vi "HowdyArcade.vi"(7 "Negate Right input (true)":bool=TRUE, 9 "forward":dbl format="%#_13g", 10 "right":dbl format="%#_13g") -> (1 "right_wheel":dbl format="%#_13g", 2 "left_wheel":dbl format="%#_13g")   [LabVIEW 2019, in "DriveOld.lvlib" / "Drive.lvclass"]
doc: "This takes a forward value and a turn value (typically from a joystick) and mixes the inputs to produce a left wheel and a right wheel speed (typically used for a tank robot setup). This preserves constant rate of turn regardless of forward demand."
uses:
  Drive.lvclass
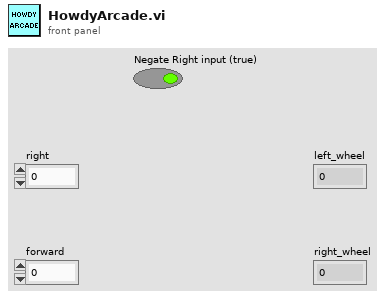
[diagram p1: front panel]
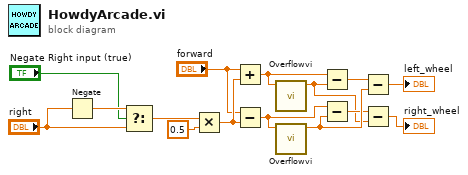
[diagram p0: block diagram]
diagram:
  n1 = Negate(x="right") -> (-x=w4:dbl)
  n2 = Select(t=w4, s="Negate Right input (true)", f="right") -> (s? t:f=w2:dbl)
  n3 = Multiply(x=w2, y=0.5) -> (x*y=w14:dbl)
  n4 = Add(x="forward", y=w14) -> (x+y=w12:dbl)
  n5 = Subtract(x="forward", y=w14) -> (x-y=w9:dbl)
  n6 = call "Overflowvi.vi"("value"=w12) -> ("overflow"=w6:dbl)  [unwired: 10 in]
  n7 = call "Overflowvi.vi"("value"=w9) -> ("overflow"=w8:dbl)  [unwired: 10 in]
  n8 = Subtract(x=w12, y=w6) -> (x-y=w11:dbl)
  n9 = Subtract(x=w9, y=w8) -> (x-y=w7:dbl)
  n10 = Subtract(x=w11, y=w8) -> (x-y=→"left_wheel":dbl)
  n11 = Subtract(x=w7, y=w6) -> (x-y=→"right_wheel":dbl)
